vi "Save Settings To Non-Volatile Memory.vi"(4 "error in (no error)":errorcluster, 7 "VISA resource name":refnum<visa-resource-name>) -> (0 "error out":errorcluster, 3 "VISA resource name out":refnum<visa-resource-name>)   [LabVIEW 2012, in "Newport ESP301.lvlib"]
doc: "This command is used to save system and axis configuration settings from RAM to non-volatile flash memory. It should be used after modifying system and/or axis parameters and settings to assure that the new data will not be lost when the controller is powered off.\nNote:\nUser programs created with EP command are automatically saved to non-volatile memory."
uses:
  Newport ESP301.lvlib
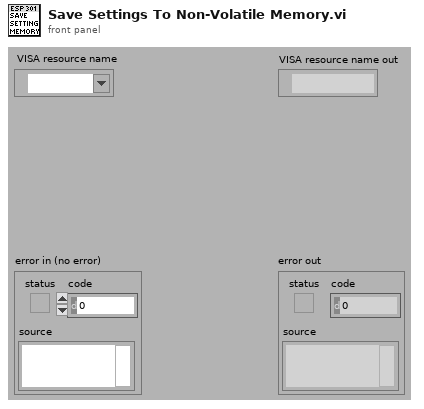
[diagram p1: front panel]
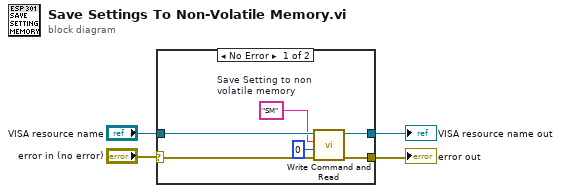
[diagram p0: block diagram]
diagram:
  n1 = case shown="No Error" "error in (no error)" {
    selector: "error in (no error)" -> [w7 w12]
    tunnel: [w9 w12] -> w4
    tunnel: "VISA resource name" -> [w10 w11]
    tunnel: [w8 w11] -> w3
    frame No Error {
      w5 = "SM"  # Save Setting to non  volatile memory
      n2 = call "Write Command and Read.vi"("error in (no error)"=w7, "Bytes to read (100)"=u32 0, "Command"=w5, "VISA resource name"=w10) -> ("error out"=w9:errorcluster, "VISA resource name out"=w8:refnum<visa-resource-name>)  [unwired: 1 in, 3 out]
    }
    frame Error {
    }
  }
  "error out" <- w4
  "VISA resource name out" <- w3
